vi "Initialise montage gen.vi"(0 "ExperimentPath":path, 2 "Channel":i32, 4 "First init.":bool, 8 "Output file path":path=path "C:/Users/Teo/Desktop/UCL Datasets/160915_13_48_57 FunctAcq-6 patches", 9 "Frames Per Second":u32=34, 11 "Number of rows to generate":i32=6) -> (14 "Cancel":bool, 15 "Experiment Parameters":T1, 17 "Output file ref":T2, 19 "error out":errorcluster)   [LabVIEW 2017]
uses:
  Prototyping/Patch data preview/Typedefs/Patch viewer states.ctl
  <vilib>/vision/Avi.llb/IMAQ AVI2 Refnum.ctl
  Typedefs/Experiment Parameters.ctl
  Prototyping/Patch data preview/Typedefs/Patch viewer internal cluster.ctl
  <vilib>/vision/Image Controls.llb/IMAQ Image.ctl
  Typedefs/Read Write Enum.ctl
  Functional Imaging Viewer/SubVIs/Experiment header interface/Typedefs/Header file sections.ctl
  Functional Imaging Viewer/SubVIs/Experiment header interface/Typedefs/Header file actions.ctl
  Globals/gl_8-bit montage window ctrl refs.vi
panel:
  out "Next state":T3
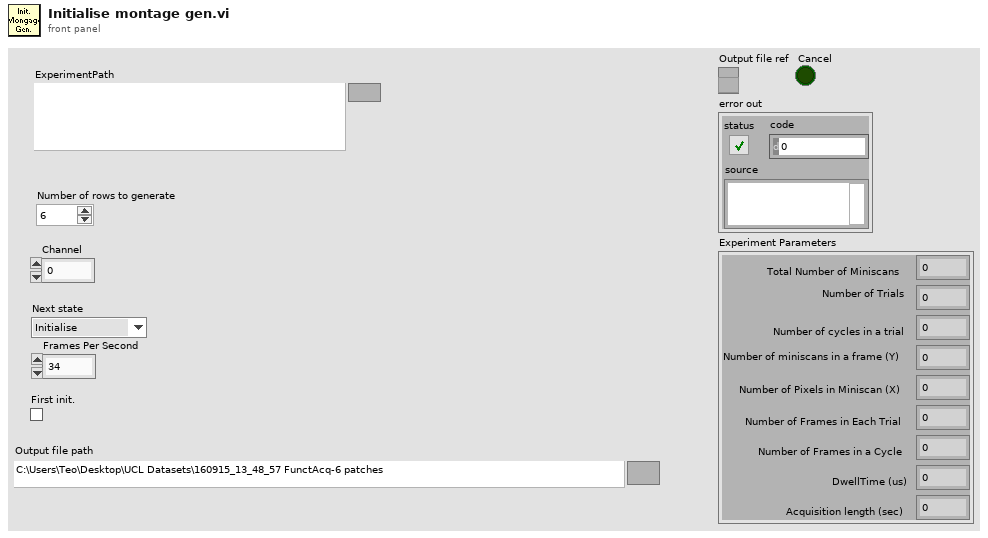
[diagram p1: front panel]
types:
  T1 = typedef "Experiment Parameters.ctl" = cluster{"Total Number of Miniscans":i32, "Number of Trials":i32, "Number of cycles in a trial":i32, "Number of miniscans in a frame (Y)":i32, "Number of Pixels in Miniscan (X)":i32, "Number of Frames in Each Trial":i32, "Number of Frames in a Cycle":i32, "DwellTime (us)":dbl, "Acquisition length (sec)":dbl}
  T2 = typedef "IMAQ AVI2 Refnum.ctl" = refnum<k20>
  T3 = typedef "Patch viewer states.ctl" = enum16{"Initialise", "Refresh", "Idle", "Error"}
  T4 = typedef "8-bit video export window ctrl refs.ctl" = cluster{"This VI":refnum<vi>, "Add speed data":refnum<vi>, "Add camera videos":refnum<vi>, "Stop button":refnum<vi>, "Camera Video Adjustments":refnum<vi>, "Microscope Image Adjustments":refnum<vi>, "Execute":refnum<vi>, "Codec":refnum<vi>, "Channel to load":refnum<vi>, "Speed graph behaviour":refnum<vi>, "Include speed graph":refnum<vi>, "Number of rows to generate":refnum<vi>, "Path":refnum<vi>}
  T5 = typedef "Header file actions.ctl" = enum16{"Create", "Open", "Read All", "Read Section", "Write All", "Write Section", "Close"}
  T6 = typedef "Header file sections.ctl" = enum16{"ALL SECTIONS", "LOGIN", "GLOBAL PARAMETERS", "IMAGING MODES", "TIME SERIES", "MOTOR Z-STACK", "AOL Z-STACK", "FUNCTIONAL IMAGING", "MOVEMENT CORRECTION", "CALIBRATION", "STATISTICS", "BIOLOGY INFORMATION"}
  T7 = typedef "Read Write Enum.ctl" = enum16{"Read", "Write"}
  T8 = typedef "Patch viewer internal cluster.ctl" = cluster{"Image ref":T9, "Coordinates of montage positions":cluster{"X\n\nY":i32[]}[], "TDMS refs":refnum<k34>[], "Frames info":cluster{"Frame numbers used":i32[], "Frame position index":i32[]}, "Number of trials":i32, "Cycles in single trial":i32, "Total number of cycles":i32, "Number of patches":i32, "Pixels in a cycle":i32, "Patches info array":cluster{"Pixels in a patch":i32, "X size of patch":i32, "Y size of patch":i32}[], "error":errorcluster}
  T9 = typedef "IMAQ Image.ctl" = refnum<image>
  T10 = cluster{"Pixels in a patch":i32, "X size of patch":i32, "Y size of patch":i32}
  T11 = cluster{"Frame numbers used":i32[], "Frame position index":i32[]}
  T12 = typedef "Header parameters cluster-ALL.ctl" = cluster{"LOGIN":T13, "GLOBAL PARAMETERS":T14, "IMAGING MODES":T16, "TIME SERIES":T17, "MOTOR Z-STACK ":T20, "AOL Z-STACK":T21, "FUNCTIONAL IMAGING":T22, "MOVEMENT CORRECTION":T26, "CALIBRATION":T28, "STATISTICS":T29, "BIOLOGY INFORMATION":T30}
  T13 = typedef "Header params -Login.ctl" = cluster{"User":string, "Profile":string, "Software Version":string, "Experiment Date Time":timestamp}
  T14 = typedef "Header params-Global Parameters.ctl" = cluster{"MicroscopeID":string, "Microscope Type":string, "Objective":string, "Field of View (um)":dbl, "Fill time (us)":dbl, "Experiment Type":T15, "Stimuli Trigger":bool, "Speed Logging":bool}
  T15 = typedef "Experiment Type.ctl" = enum16{"In vivo", "In vitro", "Testing", "Calibration", "Other"}
  T16 = typedef "Header params-Imaging Modes.ctl" = cluster{"Time Series":bool, "Motor Zstack":bool, "AOL Zstack":bool, "Functional Imaging":bool}
  T17 = typedef "Header params-Time Series.ctl" = cluster{"Basic Image meta data":T18, "AOL z":dbl}
  T18 = typedef "Header params-Basic image meta data.ctl" = cluster{"Wavelength (nm)":dbl, "# averaged frames":dbl, "laser power (%)":dbl, "Pockels":dbl, "pixel dwell time (us)":dbl, "pmt 1":dbl, "pmt 2":dbl, "back apperture":dbl, "zoom":dbl, "field of view":dbl, "Frame Size":T19, "AOL x centre":dbl, "AOL y centre":dbl, "Stage x position":dbl, "Stage y position":dbl, "Stage z position":dbl}
  T19 = typedef "Frame Size.ctl" = u16
  T20 = typedef "Header params-Motor Z-stack.ctl" = cluster{"Hdr Basic Image meta data":T18, "Z Start":dbl, "Z Stop":dbl, "No of Planes":i32}
  T21 = typedef "Header params-AOL Z-stack.ctl" = cluster{"Hdr Basic Image meta data":T18, "Z Start":dbl, "Z Stop":dbl, "No of Planes":i32}
  T22 = typedef "Header params-Functional Imaging.ctl" = cluster{"Functional Mode":T23, "Pockels Modulation":bool, "Number of pois":dbl, "Number of miniscans":dbl, "Number of cycles":dbl, "Number of trials":dbl, "Miniscan dwell time per pixel (us)":dbl, "Number of pixels in miniscan":dbl, "poi dwell time":dbl, "Rectangle ROI length":dbl, "Rectangle ROI height":dbl, "AOL Mode":T24, "Plane Mode":T25, "video length (sec)":dbl, "Frame rate (fps)":dbl, "Stimuli Timing (usec)":dbl, "Acquisition Length":dbl, "Basic Image meta data":T18, "Z Start (um)":dbl, "Z Stop (um)":dbl}
  T23 = typedef "Functional Mode.ctl" = enum16{"Point", "Line", "Patch", "Plane", "Volume"}
  T24 = typedef "AOL modes.ctl" = enum16{"Raster", "Structural", "Pointing", "Mini Scan", "Alignment"}
  T25 = typedef "Plane Mode.ctl" = u16
  T26 = typedef "Header params-Movement correction.ctl" = cluster{"Movement Correction":bool, "Axial Reference":bool, "Reference X Pixels":dbl, "Reference Y Pixels":dbl, "Reference Source":T27, "Reference dwell time (us)":dbl, "Number of Z lines":dbl, "Size of Z pixels":dbl, "Axial Pixels":dbl, "Reference Zoom":dbl, "Reference Average":dbl, "Proportional Scale":dbl, "Integral Scale":dbl, "Proportional Scale Z":dbl, "Integral Scale Z":dbl, "Scan Interval":dbl, "Ref Plot Refresh Rate":dbl}
  T27 = typedef "Reference source.ctl" = enum16{"Green channel", "Red channel"}
  T28 = typedef "Header params-Calibration Setup.ctl" = cluster{"Pockels Calibration File":path, "Calibration_ini file":path, "Setup_ini file":path}
  T29 = typedef "Header params-statistics.ctl" = cluster{"Z-stack duration (sec)":dbl, "Number of acquired data-points":dbl, "Acquisition time (ms)":dbl, "Number of acquired frames":dbl}
  T30 = typedef "Biology Information.ctl" = cluster{"Animal Code or Name":string, "Animal DoB":string, "Animal Age":string, "Animal Sex":string, "Animal Weight":string, "Date of Injection":string, "Date of Implant":string, "Site of Injection":string, "Animal Ear Notch":string, "AAV constructs":string, "Genetic background":string, "Optical reporter":string, "Region of brain imaged":string, "Other \ncomments":string}
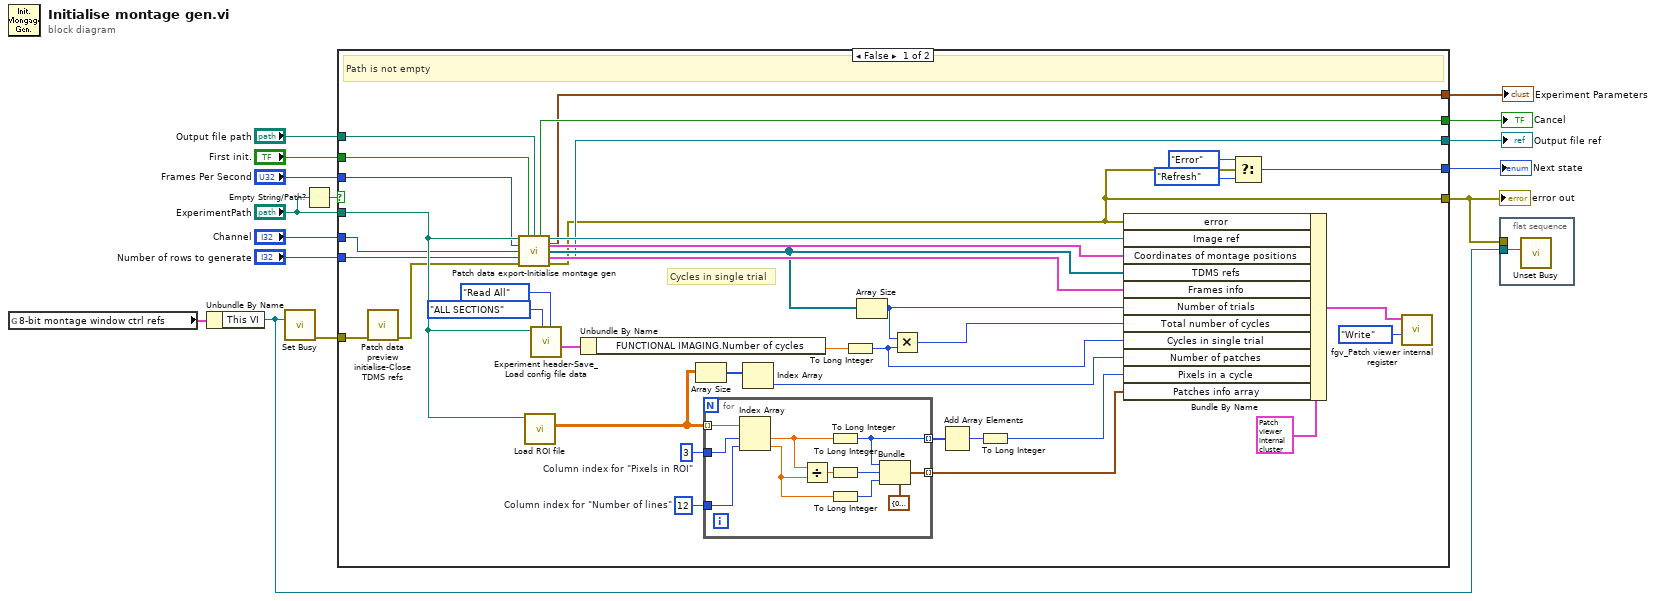
[diagram p0: block diagram]
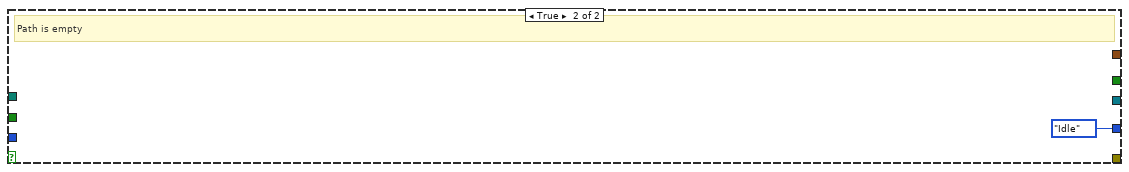
[diagram p2: hidden frame]
diagram:
  n1 = global read "gl_8-bit montage window ctrl refs.vi" "8-bit montage window ctrl refs"() -> (w6:T4)
  n2 = Unbundle By Name(w6) -> ("This VI"=w3:refnum<vi>)
  n3 = call <vilib>:"Set Busy.vi"("VI reference (current VI)"=w3) -> ("error out"=w5:errorcluster)  [unwired: 9 in, 1 out]
  n4 = Empty String/Path?(string/path="ExperimentPath") -> (empty?=w14:bool)
  n5 = case shown="False" w14 {
    tunnel: "ExperimentPath" -> [w53 _]
    tunnel: "Number of rows to generate" -> [w28 _]
    tunnel: [w36 Patch_viewer_states."Idle" ("States")] -> w15
    tunnel: [w27 _] -> w11
    tunnel: [w26 _] -> w4
    tunnel: [w25 _] -> w10
    tunnel: [w24 _] -> w9
    tunnel: "Frames Per Second" -> [w23 _]
    tunnel: "Channel" -> [w22 _]
    tunnel: w5 -> [w21 _]
    tunnel: "First init." -> [w20 _]
    tunnel: "Output file path" -> [w19 _]
    frame False {
      w48 = 3  # Column index for "Pixels in ROI"
      w47 = 12  # Column index for "Number of lines"
      # "Cycles in single trial"
      # "Path is not empty"
      n6 = call "Patch data preview initialise-Close TDMS refs.vi"("error in"=w21) -> ("error out (no error)"=w35:errorcluster)  [unwired: 10 in]
      n7 = call "Patch data export-Initialise montage gen.vi"("ExperimentPath"=w53, "First init."=w20, "Output file path"=w19, "Frames Per Second"=w23, "Channel"=w22, "Number of rows to generate"=w28, "error in (no error)"=w35) -> ("Experiment Parameters"=w24:T1, "Image ref (Montage)"=w41:T9, "Coordinates of montage positions"=w42:cluster{"X\n\nY":i32[]}[], "TDMS references(All Trials)"=w34:refnum<k34>[], "Frames info"=w43:T11, "Cancel"=w25:bool, "AVI Refnum"=w27:T2, "error out"=w26:errorcluster)  [unwired: 1 in]
      n8 = call "Load ROI file.vi"("Experiment data folder path"=w53) -> ("ROI Data (header removed)"=w45:dbl[][])  [unwired: 7 in, 3 out]
      n9 = call "Experiment header-Save_Load config file data.vi"("Header file actions"=Header_file_actions."Read All", "Header file sections"=Header_file_sections."ALL SECTIONS", "Experiment data folder path"=w53) -> ("All header parameters out"=w46:T12)  [unwired: 7 in, 1 out]
      n10 = Unbundle By Name(w46) -> ("FUNCTIONAL IMAGING.Number of cycles"=w49:dbl)
      n11 = Array Size(array=w45) -> (size(s)=w50:i32[])
      n12 = for {
        tunnel: w45 -> [w64] mode=indexing
        tunnel: w48 -> [w63]
        tunnel: w47 -> [w62]
        tunnel: [w59] -> w16 mode=indexing
        tunnel: [w54] -> w52 mode=indexing
        n13 = Index Array(array=w64, index #1=w63, index #2=w62) -> (element #1=w58:dbl, element #2=w60:dbl)
        n14 = Divide(x=w58, y=w60) -> (x/y=w61:dbl)
        n15 = To Long Integer(number=w58) -> (32bit integer=w54:i32)
        n16 = To Long Integer(number=w61) -> (32bit integer=w55:i32)
        n17 = To Long Integer(number=w60) -> (32bit integer=w56:i32)
        n18 = Bundle(cluster=T10 {"Pixels in a patch"=0, "X size of patch"=0, "Y size of patch"=0}, "Pixels in a patch"=w54, "X size of patch"=w55, "Y size of patch"=w56) -> (w59:T10)
      }
      n19 = Index Array(array=w50) -> (element=w39:i32)  [unwired: 1 in]
      n20 = To Long Integer(number=w49) -> (32bit integer=w33:i32)
      n21 = Array Size(array=w34) -> (size(s)=w32:i32)
      n22 = Multiply(x=w32, y=w33) -> (x*y=w29:i32)
      n23 = Add Array Elements(numeric array=w52) -> (sum=w51:i32)
      n24 = To Long Integer(number=w51) -> (32bit integer=w40:i32)
      n25 = Bundle By Name(cluster=T8 {"Image ref"=refnum, "Coordinates of montage positions"=[], "TDMS refs"=[], "Frames info"={"Frame numbers used"=[], "Frame position index"=[]}, "Number of trials"=0, "Cycles in single trial"=0, "Total number of cycles"=0, "Number of patches"=0, "Pixels in a cycle"=0, "Patches info array"=[], "error"={"status"=FALSE, "code"=0, "source"=""}} ("Register cluster"), "error"=w26, "Image ref"=w41, "Coordinates of montage positions"=w42, "TDMS refs"=w34, "Frames info"=w43, "Number of trials"=w32, "Total number of cycles"=w29, "Cycles in single trial"=w33, "Number of patches"=w39, "Pixels in a cycle"=w40, "Patches info array"=w16) -> (w30:T8)
      n26 = Select(t=Patch_viewer_states."Error" ("States"), s=w26, f=Patch_viewer_states."Refresh" ("States")) -> (s? t:f=w36:T3)
      n27 = call "fgv_Patch viewer internal register.vi"("Function"=Read_Write_Enum."Write", "Registered setup"=w30) -> ()  [unwired: 9 in, 1 out]
    }
    frame True {
      # "Path is empty"
    }
  }
  "Next state" <- w15
  "Output file ref" <- w11
  "error out" <- w4
  "Cancel" <- w10
  "Experiment Parameters" <- w9
  n28 = flat-sequence {
    tunnel: w4 -> [_]
    tunnel: w3 -> [w66]
    frame #0 {
      n29 = call <vilib>:"Unset Busy.vi"("VI reference (current VI)"=w66) -> ()  [unwired: 10 in, 1 out]
    }
  }
